vi "hardware_close_hardware.vi"(8 "error in (no error)":errorcluster, 11 "thorlabs_kinesis in":refnum<class "thorlabs_kinesis.lvclass">) -> (0 "error out":errorcluster, 3 "thorlabs_kinesis out":refnum<class "thorlabs_kinesis.lvclass">)   [LabVIEW 2015, in "thorlabs_kinesis.lvclass"]
uses:
  thorlabs_kinesis.lvclass
  thorlabs_kinesis.lvclass/thorlabs_kinesis.ctl
  thorlabs_drivers/Thorlabs.MotionControl.Benchtop.Piezo.dll
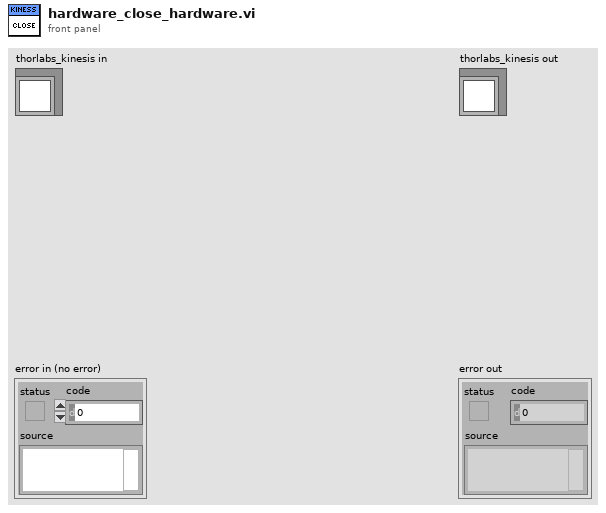
[diagram p1: front panel]
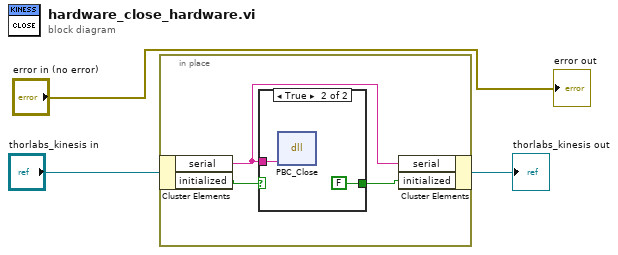
[diagram p0: block diagram]
diagram:
  n1 = in-place {
    n2 = in-place-cluster #1("thorlabs_kinesis in") -> ("serial"=w4:string, "initialized"=w6:bool)
    n3 = case shown="True" w6 {
      selector: w6 -> [w7 _]
      tunnel: w4 -> [_ w9]
      tunnel: [w7 FALSE] -> w5
      frame False {
      }
      frame True {
        n4 = dll-call lib="C:/Users/MX-Microscope/Documents/LabVIEW Data/lvoop_campus_2018/Stage Class/Thorlabs Kinesis/thorlabs_drivers/Thorlabs.MotionControl.Benchtop.Piezo.dll" fn="PBC_Close"("serial"=w9) -> ()  [unwired: 5 in, 2 out]
      }
    }
    n5 = in-place-cluster #1("serial"=w4, "initialized"=w5) -> (→"thorlabs_kinesis out":refnum<class "thorlabs_kinesis.lvclass">)
  }
  "error out" <- "error in (no error)"
